vi "Get_Frames.vi"(8 "error in (no error)":errorcluster, 11 "Avantes in":refnum<class "Avantes.lvclass">) -> (0 "error out":errorcluster, 2 "Frames":i32=-5000, 3 "Avantes out":refnum<class "Avantes.lvclass">)   [LabVIEW 2020, in "Avantes.lvclass"]
uses:
  <instrlib>/Classes/CCD/Avantes/Avantes.lvclass
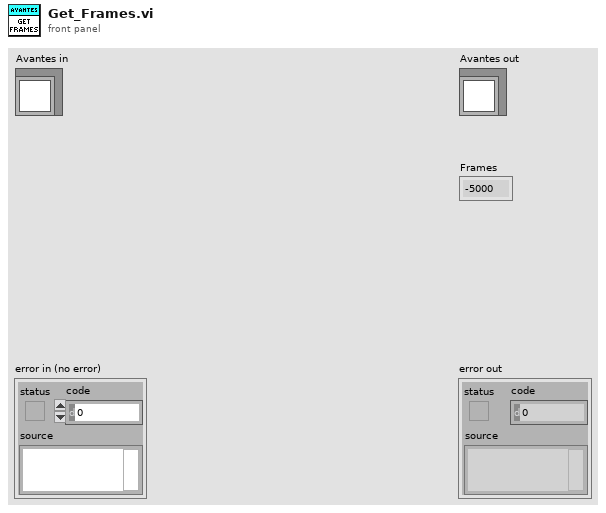
[diagram p1: front panel]
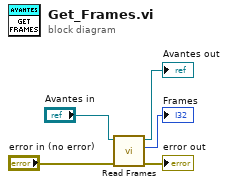
[diagram p0: block diagram]
diagram:
  n1 = call-dynamic "Read Frames.vi"("error in (no error)"="error in (no error)", "Avantes in"="Avantes in") -> ("error out"=→"error out":errorcluster, "Frames"=→"Frames":i32, "Avantes out"=→"Avantes out":refnum<class "Avantes.lvclass">)  [unwired: 7 in]
